vi "Sort Complex Numbers (Magnitude).vi"(10 "Order":enum16{"Ascending", "Descending"}(ring), 11 "Complex Numbers":cdb[](array[numeric]) format="%#.6g") -> (0 "error":i32, 2 "Sorted Index":i32[](array[numeric]), 3 "Sorted Complex Numbers":cdb[](array[numeric]) format="%#.6g")   [LabVIEW 2017, in "NI_AALPro.lvlib"]
doc: "Sorts an array of complex numbers in ascending or descending order with respect to their magnitudes."
uses:
  <vilib>/Analysis/NI_AALPro.lvlib
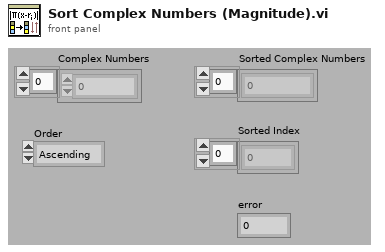
[diagram p1: front panel]
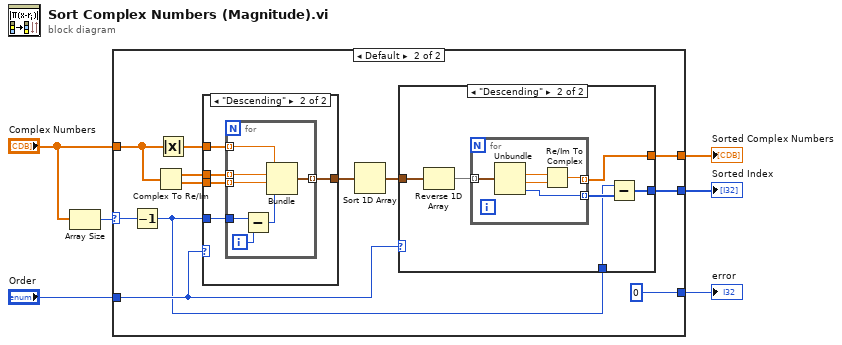
[diagram p0: block diagram]
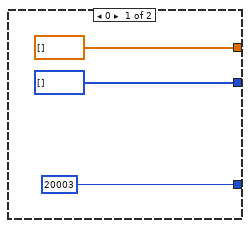
[diagram p2: hidden frame]
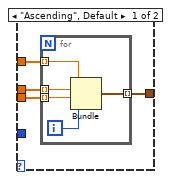
[diagram p3: hidden frame]
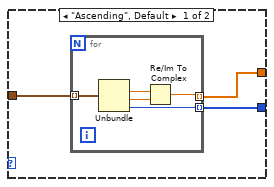
[diagram p4: hidden frame]
diagram:
  n1 = Array Size(array="Complex Numbers") -> (size(s)=w3:i32)
  n2 = case shown="Default" w3 {
    selector: w3 -> [_ w14]
    tunnel: "Complex Numbers" -> [_ w18]
    tunnel: [i32[] [] w12] -> w6
    tunnel: [cdb[] [] ("CDB") w11] -> w5
    tunnel: "Order" -> [_ w17]
    tunnel: [20003 ("empty array") 0 ("empty array")] -> w1
    frame 0 {
    }
    frame Default {
      n3 = Decrement(x=w14) -> (x-1=w10:i32)
      n4 = Complex To Re/Im(x + iy=w18) -> (x=w16:dbl[], y=w15:dbl[])
      n5 = Absolute Value(x=w18) -> (abs(x)=w21:dbl[])
      n6 = case shown="\"Descending\"" w17 {
        tunnel: w21 -> [w25 w35]
        tunnel: [w24 w34] -> w20
        tunnel: w16 -> [w23 w33]
        tunnel: w15 -> [w22 w32]
        tunnel: w10 -> [_ w31]
        frame "Ascending", Default {
          n7 = for {
            tunnel: [w30] -> w24 mode=indexing
            tunnel: w25 -> [w29] mode=indexing
            tunnel: w23 -> [w28] mode=indexing
            tunnel: w22 -> [w27] mode=indexing
            i -> [w26]
            n8 = Bundle(w29, w28, w27, w26) -> (w30:cluster{dbl, dbl, dbl, i32})  [unwired: 1 in]
          }
        }
        frame "Descending" {
          n9 = for {
            tunnel: [w42] -> w34 mode=indexing
            tunnel: w35 -> [w41] mode=indexing
            tunnel: w33 -> [w40] mode=indexing
            tunnel: w32 -> [w39] mode=indexing
            tunnel: w31 -> [w37]
            i -> [w36]
            n10 = Subtract(x=w37, y=w36) -> (x-y=w38:i32)
            n11 = Bundle(w41, w40, w39, w38) -> (w42:cluster{dbl, dbl, dbl, i32})  [unwired: 1 in]
          }
        }
      }
      n12 = Sort 1D Array(array=w20) -> (sorted array=w19:cluster{dbl, dbl, dbl, i32}[])
      n13 = case shown="\"Descending\"" w17 {
        tunnel: w19 -> [w45 w56]
        tunnel: [w44 w53] -> w12
        tunnel: [w43 w54] -> w11
        tunnel: w10 -> [_ w51]
        frame "Ascending", Default {
          n14 = for {
            tunnel: w45 -> [w50] mode=indexing
            tunnel: [w47] -> w43 mode=indexing
            tunnel: [w46] -> w44 mode=indexing
            n15 = Unbundle(w50) -> (w48:dbl, w49:dbl, w46:i32)  [unwired: 1 out]
            n16 = Re/Im To Complex(1:w49, 2:w48) -> (0:w47:cdb)
          }
        }
        frame "Descending" {
          n17 = Reverse 1D Array(array=w56) -> (reversed array=w55:cluster{dbl, dbl, dbl, i32}[])
          n18 = for {
            tunnel: w55 -> [w61] mode=indexing
            tunnel: [w58] -> w54 mode=indexing
            tunnel: [w57] -> w52 mode=indexing
            n19 = Unbundle(w61) -> (w59:dbl, w60:dbl, w57:i32)  [unwired: 1 out]
            n20 = Re/Im To Complex(1:w60, 2:w59) -> (0:w58:cdb)
          }
          n21 = Subtract(x=w51, y=w52) -> (x-y=w53:i32[])
        }
      }
    }
  }
  "Sorted Index" <- w6
  "Sorted Complex Numbers" <- w5
  "error" <- w1
